vi "PXI-Reset Devices.vi"(8 "error in":errorcluster) -> (0 "error out":errorcluster)   [LabVIEW 2020]
uses:
  <resource>/objmgr/daqmx.rc
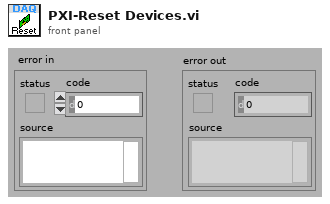
[diagram p1: front panel]
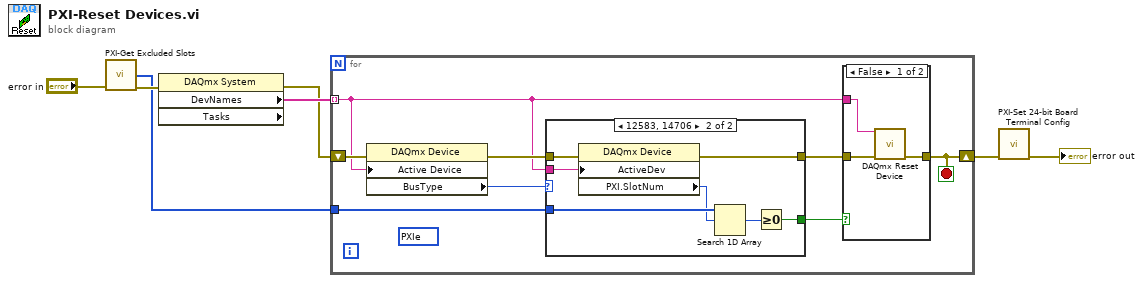
[diagram p0: block diagram]
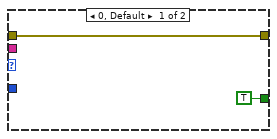
[diagram p2: hidden frame]
diagram:
  n1 = call "PXI-Get Excluded Slots.vi"("error in (no error)"="error in") -> ("excluded slots"=w3:i32[], "error out"=w4:errorcluster)  [unwired: 13 in]
  n2 = property class="DAQmx System" props=["DevNames", "Tasks"](error in=w4) -> (error out=w6:errorcluster, "DevNames"=w7:tag[])  [unwired: 1 in, 2 out]
  n3 = for {
    tunnel: w7 -> [w8] mode=indexing
    shift-right: [w9] -> w2
    shift-left: w6 -> [w12]
    tunnel: w3 -> [w15]
    stop <- w9 stop-if-true
    (unwired) 14706 items=["PCI"=12582, "PCIe"=13612, "PXI"=12583, "PXIe"=14706, "SCXI"=12584, "SCC"=14707, "PCCard"=12585, "USB"=12586, "CompactDAQ"=14637, "TCP/IP"=14828, "Unknown"=12588, "SwitchBlock"=15870] ("BusType")
    n4 = property class="DAQmx Device"(error in=w12, "Active Device"=w8) -> (error out=w11:errorcluster, "BusType"=w10:i32)  [unwired: 1 in, 1 out]
    n5 = case shown="12583, 14706" w10 {
      tunnel: w15 -> [_ w24]
      tunnel: [TRUE w22] -> w14
      tunnel: [w17 w21] -> w13
      tunnel: w11 -> [w17 w20]
      tunnel: w8 -> [_ w18]
      frame 0, Default {
      }
      frame 12583, 14706 {
        n6 = property class="DAQmx Device"(error in=w20, "ActiveDev"=w18) -> (error out=w21:errorcluster, "PXI.SlotNum"=w19:u32)  [unwired: 1 in, 1 out]
        n7 = Search 1D Array(1D array=w24, element=w19) -> (index of element=w23:i32)  [unwired: 1 in]
        n8 = Greater Or Equal To 0?(x=w23) -> (x >= 0?=w22:bool)
      }
    }
    n9 = case shown="False" w14 {
      tunnel: [w27 w28] -> w9
      tunnel: w13 -> [w26 w28]
      tunnel: w8 -> [w25 _]
      frame False {
        n10 = call <vilib>:"DAQmx Reset Device.vi"("device in"=w25, "error in"=w26) -> ("error out"=w27:errorcluster)  [unwired: 13 in]
      }
      frame True {
      }
    }
  }
  n11 = call "PXI-Set 24-bit Board Terminal Config.vi"("error in (no error)"=w2) -> ("error out"=→"error out":errorcluster)  [unwired: 14 in]
